vi "ReadAllVip.vi"(8 "error in (no error)":errorcluster, 11 "Cartella VIP locale":path) -> (0 "error out":errorcluster, 3 "LocalVip":T1[](array[typedef]))   [LabVIEW 2019, in "ByteLVDevEnv.lvlib"]
uses:
  ByteLVDevEnv.lvlib
  TypeDefs/AllLibraries.ctl
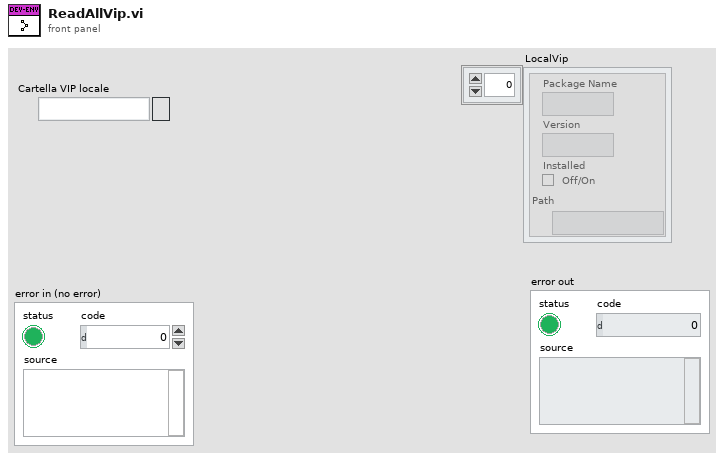
[diagram p1: front panel]
types:
  T1 = typedef "ByteLVDevEnv.lvlib/AllLibraries.ctl" = cluster{"Package Name":string, "Version":string, "Installed":bool, "Path":path}
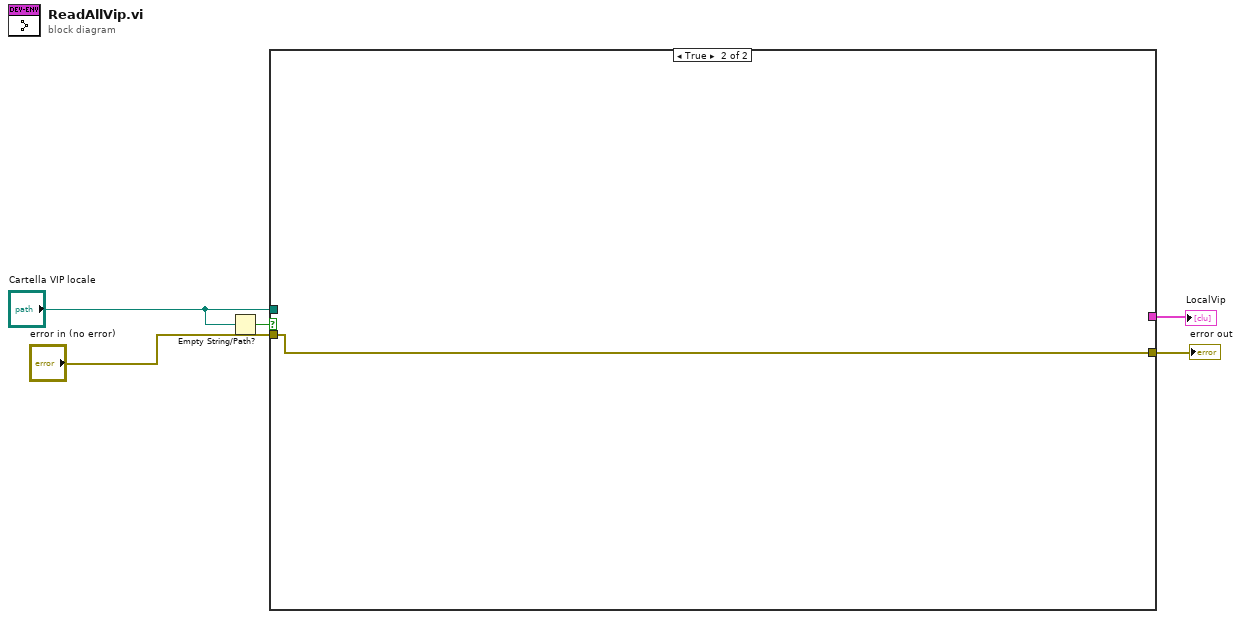
[diagram p0: block diagram]
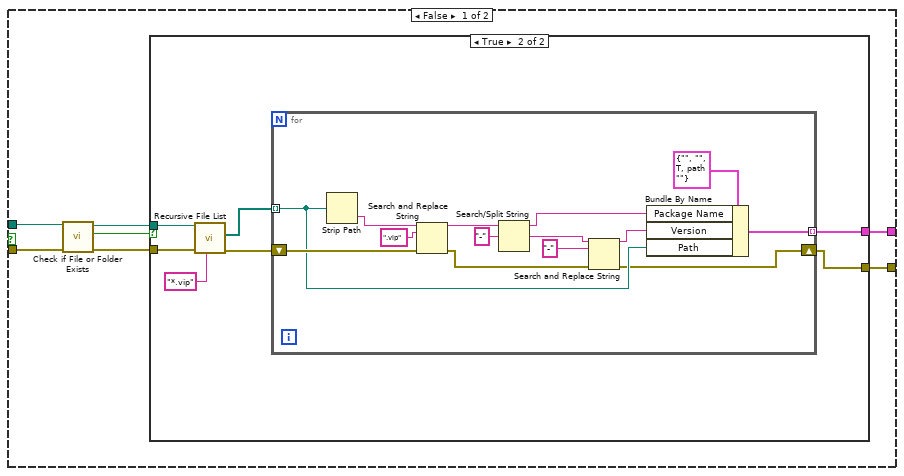
[diagram p2: hidden frame]
diagram:
  n1 = Empty String/Path?(string/path="Cartella VIP locale") -> (empty?=w2:bool)
  n2 = case shown="True" w2 {
    tunnel: "Cartella VIP locale" -> [w10 _]
    tunnel: "error in (no error)" -> [w9 w35]
    tunnel: [w7 w35] -> w4
    tunnel: [w6 _] -> w3
    frame False {
      n3 = call <vilib>:"Check if File or Folder Exists.vi"("error in (no error)"=w9, "path"=w10) -> ("error out"=w12:errorcluster, "file or folder exists?"=w8:bool, "dup path"=w11:path)  [unwired: 7 in]
      n4 = case shown="True" w8 {
        tunnel: w12 -> [w13 w17]
        tunnel: w11 -> [_ w16]
        tunnel: [w13 w15] -> w7
        tunnel: [_ w14] -> w6
        frame False {
        }
        frame True {
          n5 = call <vilib>:"Recursive File List.vi"("pattern"="*.vip", "error in (no error)"=w17, "Folder Path"=w16) -> ("error out"=w18:errorcluster, "All Files in Dir"=w19:path[])  [unwired: 4 in, 3 out]
          n6 = for {
            tunnel: w19 -> [w29] mode=indexing
            tunnel: [w28] -> w14 mode=indexing
            shift-right: [w22] -> w15
            shift-left: w18 -> [w34]
            n7 = Strip Path(path=w29) -> (name=w33:string)  [unwired: 1 out]
            n8 = Search and Replace String(input string=w33, search string=".vip" ("replace string (\"\")"), error in=w34) -> (result string=w32:string, error out=w26:errorcluster)  [unwired: 5 in, 2 out]
            n9 = Search/Split String(string=w32, search string/char (-)="-") -> (substring before match=w30:string, match + rest of string=w24:string)  [unwired: 1 in, 1 out]
            n10 = Search and Replace String(input string=w24, search string="-" ("replace string (\"\")"), error in=w26) -> (result string=w25:string, error out=w22:errorcluster)  [unwired: 5 in, 2 out]
            n11 = Bundle By Name(cluster=T1 {"Package Name"="", "Version"="", "Installed"=TRUE, "Path"=path ""}, "Package Name"=w30, "Version"=w25, "Path"=w29) -> (w28:T1)
          }
        }
      }
    }
    frame True {
    }
  }
  "error out" <- w4
  "LocalVip" <- w3
